vi "number_of_channels.vi"(8 "error in (no error)":errorcluster, 9 "Number of position channels":i32, 10 "Number of colour channels":i32) -> (0 "error IO":errorcluster, 1 "Number of colour channels":i32, 2 "Number of position channels":i32)   [LabVIEW 2010]
panel:
  in  "OK":bool
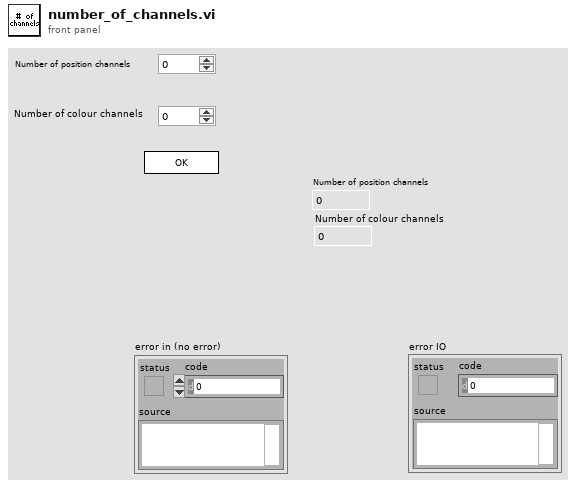
[diagram p1: front panel]
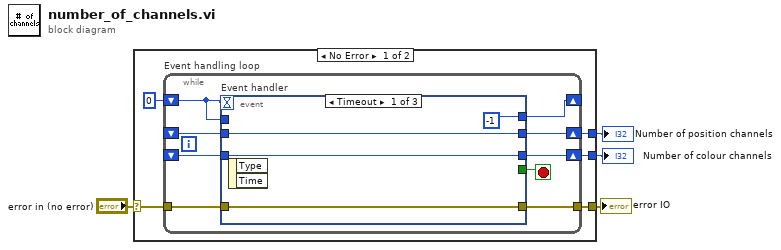
[diagram p0: block diagram]
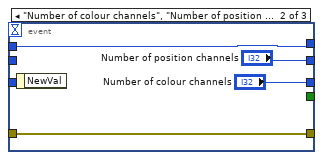
[diagram p2: hidden frame]
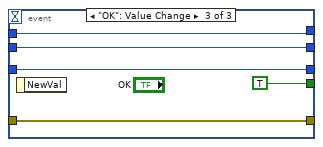
[diagram p3: hidden frame]
diagram:
  n1 = case shown="No Error" "error in (no error)" {
    selector: "error in (no error)" -> [w6 w32]
    tunnel: [w5 w32] -> w3
    tunnel: [w8 _] -> w1
    tunnel: [w7 _] -> w2
    frame No Error {
      n2 = while "Event handling loop" {
        shift-right: [w17] -> _
        shift-left: 0 -> [w18]
        shift-right: [w16] -> w7
        shift-left: _ -> [w13]
        shift-right: [w15] -> w8
        shift-left: _ -> [w14]
        tunnel: w6 -> [w11]
        tunnel: [w10] -> w5
        stop <- w12 stop-if-true
        n3 = event "Event handler" shown="[0] Timeout" {
          selector: _ -> [_ _ _]
          dyn-events: _ -> [_ _ _]
          timeout: w18 -> [_ _ _]
          tunnel: w18 -> [_ w24 w30]
          tunnel: [-1 w24 w30] -> w17
          tunnel: [w20 "Number of position channels" w29] -> w16
          tunnel: [w21 "Number of colour channels" w28] -> w15
          tunnel: w14 -> [w21 _ w28]
          tunnel: w13 -> [w20 _ w29]
          tunnel: [_ _ TRUE] -> w12
          tunnel: w11 -> [w19 w23 w27]
          tunnel: [w19 w23 w27] -> w10
          event Timeout {
            n4 = event-data() -> ()  [unwired: 1 in, 2 out]
          }
          event "Number of colour channels", "Number of position channels": Value Change {
            n5 = event-data() -> ()  [unwired: 1 in, 1 out]
          }
          event "OK": Value Change {
            n6 = event-data() -> ()  [unwired: 1 in, 1 out]
          }
        }
      }
    }
    frame Error {
    }
  }
  "error IO" <- w3
  "Number of position channels" <- w2
  "Number of colour channels" <- w1
